vi "Send_Datagram.vi"() -> ()   [LabVIEW 2018]
uses:
  Type_Def/Type_Def ControlState.ctl
panel:
  in  "Port Number":u16
  in  "IP Address target":string
  in  "Team ID":u8
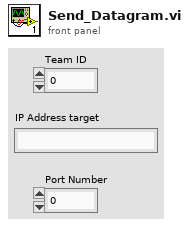
[diagram p1: front panel]
types:
  T1 = typedef "Type_Def ControlState.ctl" = enum16{"Blank", "Systems Check", "Idle", "Ready", "Pushing", "CrawlingPrecharge", "Braking", "Fault", "Boot Up", "Unpowered", "Crawling", "Shutdown", "Service Push", "Service Wait", "Vent", "Precharge"}
  T2 = cluster{"Forward":bool, "Low Side":bool, "Precharge":bool, "High Side":bool, "Digital Out 5":bool, "Digital Out 6":bool, "Digital Out 7 ":bool, "24 Power":bool, "Tank Valve ":bool, "Brake Valve":bool, "Pump":bool, "Digital Out 1 ":bool, "Digital Out 2":bool, "Digital Out 3":bool, "Digital Out 4 ":bool, "Reverse":bool}
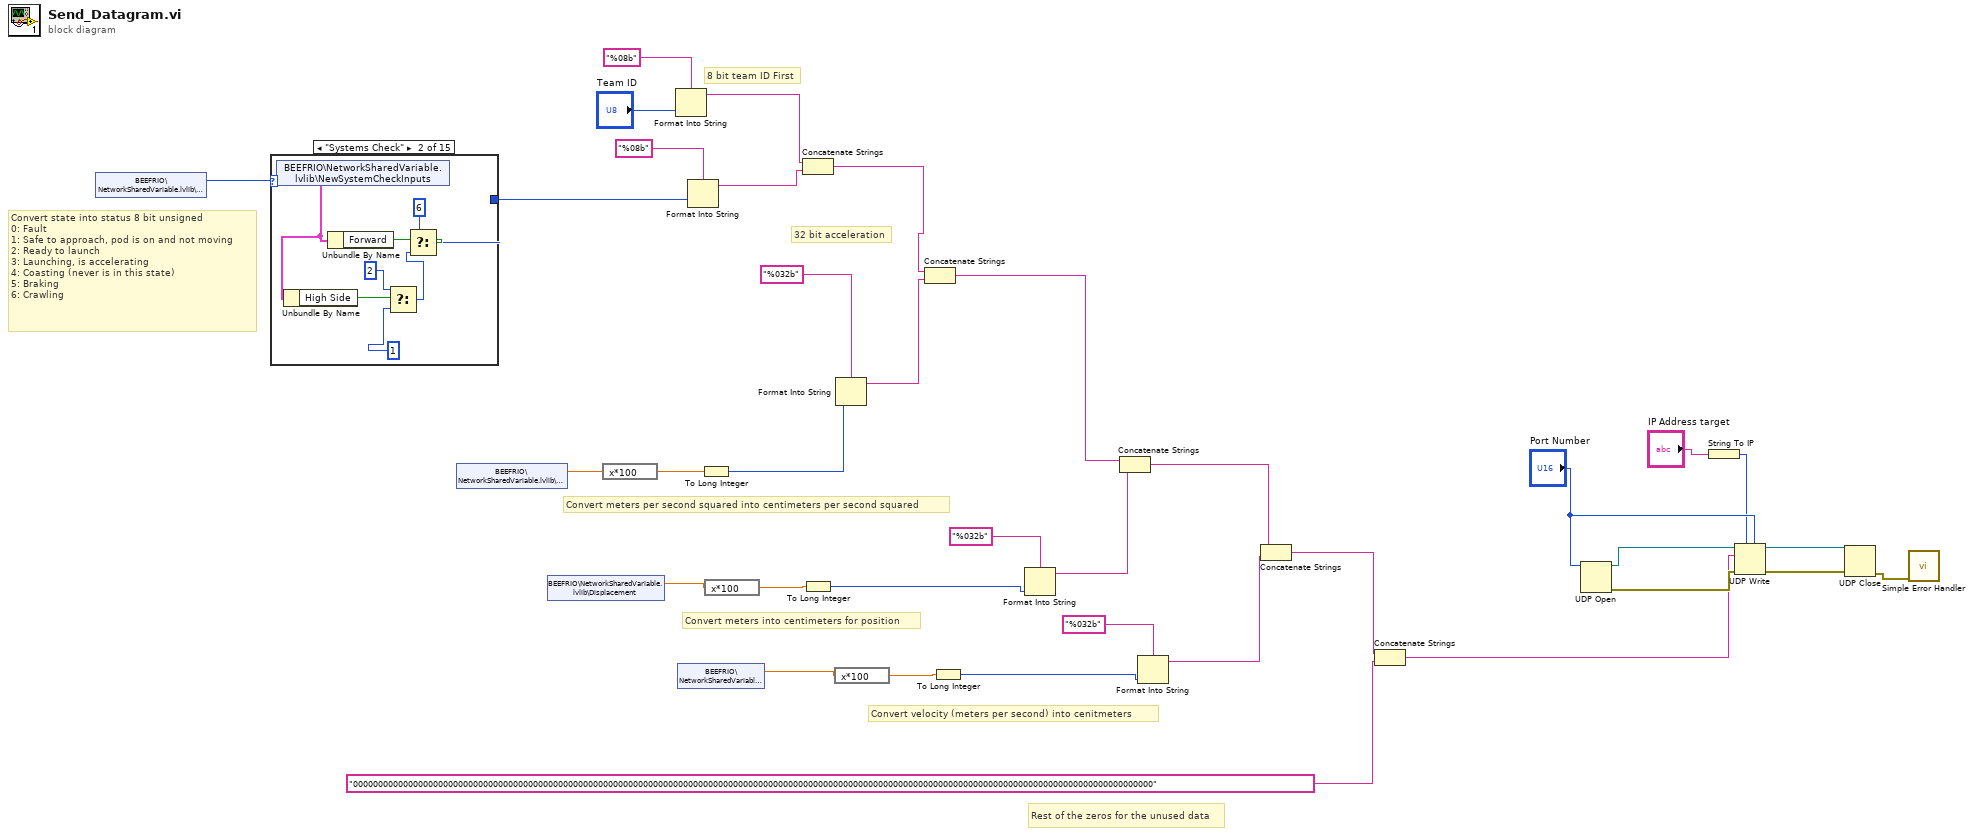
[diagram p0: block diagram]
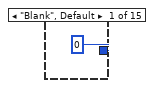
[diagram p2: hidden frame]
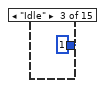
[diagram p3: hidden frame]
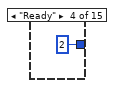
[diagram p4: hidden frame]
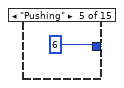
[diagram p5: hidden frame]
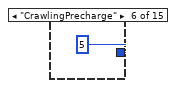
[diagram p6: hidden frame]
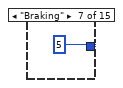
[diagram p7: hidden frame]
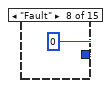
[diagram p8: hidden frame]
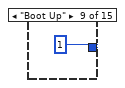
[diagram p9: hidden frame]
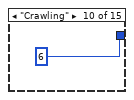
[diagram p10: hidden frame]
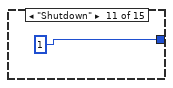
[diagram p11: hidden frame]
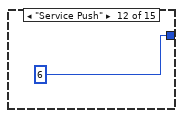
[diagram p12: hidden frame]
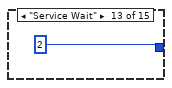
[diagram p13: hidden frame]
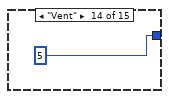
[diagram p14: hidden frame]
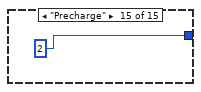
[diagram p15: hidden frame]
diagram:
  # "Rest of the zeros for the unused data"
  # "Convert velocity (meters per second) into cenitmeters"
  # "Convert meters into centimeters for position"
  # "32 bit acceleration"
  # "Convert meters per second squared into centimeters per second squared"
  # "8 bit team ID First"
  # "Convert state into status 8 bit unsigned\n0: Fault\n1: Safe to approach, pod is on and not moving\n2: Ready to launch\n3: Launching, is accelerating\n4: Coasting (never is in this state)\n5: Braking\n6: Crawling"
  n1 = shared-variable "BEEFRIO\\NetworkSharedVariable.lvlib\\CurrentState"() -> (w2:T1)  [unwired: 1 in, 1 out]
  n2 = case shown="\"Systems Check\"" w2 {
    tunnel: [u8 0 w38 u8 1 u8 2 u8 6 u8 5 u8 5 u8 0 u8 1 u8 6 u8 1 u8 6 u8 2 u8 5 u8 2] -> w1
    frame "Blank", Default {
    }
    frame "Systems Check" {
      n3 = shared-variable "BEEFRIO\\NetworkSharedVariable.lvlib\\NewSystemCheckInputs"() -> (w43:T2)  [unwired: 1 in, 1 out]
      n4 = Unbundle By Name(w43) -> ("High Side"=w42:bool)
      n5 = Unbundle By Name(w43) -> ("Forward"=w45:bool)
      n6 = Select(t=u8 2, s=w42, f=u8 1) -> (s? t:f=w39:u8)
      n7 = Select(t=u8 6, s=w45, f=w39) -> (s? t:f=w38:u8)
    }
    frame "Idle" {
    }
    frame "Ready" {
    }
    frame "Pushing" {
    }
    frame "CrawlingPrecharge" {
    }
    frame "Braking" {
    }
    frame "Fault" {
    }
    frame "Boot Up" {
    }
    frame "Crawling" {
    }
    frame "Shutdown" {
    }
    frame "Service Push" {
    }
    frame "Service Wait" {
    }
    frame "Vent" {
    }
    frame "Precharge" {
    }
  }
  n8 = shared-variable "BEEFRIO\\NetworkSharedVariable.lvlib\\Acceleration"() -> (w8:dbl)  [unwired: 1 in, 1 out]
  n9 = shared-variable "BEEFRIO\\NetworkSharedVariable.lvlib\\Displacement"() -> (w11:dbl)  [unwired: 1 in, 1 out]
  n10 = expression code="x*100"(w8) -> (w7:dbl)
  n11 = Format Into String(format string="%08b", "Team ID") -> (resulting string=w33:string)  [unwired: 2 in, 1 out]
  n12 = shared-variable "BEEFRIO\\NetworkSharedVariable.lvlib\\Velocity"() -> (w5:dbl)  [unwired: 1 in, 1 out]
  n13 = Format Into String(format string="%08b", w1) -> (resulting string=w35:string)  [unwired: 2 in, 1 out]
  n14 = To Long Integer(number=w7) -> (32bit integer=w6:i32)
  n15 = expression code="x*100"(w11) -> (w10:dbl)
  n16 = Concatenate Strings(w33, w35) -> (w30:string)
  n17 = To Long Integer(number=w10) -> (32bit integer=w9:i32)
  n18 = expression code="x*100"(w5) -> (w4:dbl)
  n19 = Format Into String(format string="%032b", w6) -> (resulting string=w29:string)  [unwired: 2 in, 1 out]
  n20 = Concatenate Strings(w30, w29) -> (w26:string)
  n21 = To Long Integer(number=w4) -> (32bit integer=w3:i32)
  n22 = Format Into String(format string="%032b", w9) -> (resulting string=w27:string)  [unwired: 2 in, 1 out]
  n23 = Concatenate Strings(w26, w27) -> (w23:string)
  n24 = Format Into String(format string="%032b", w3) -> (resulting string=w24:string)  [unwired: 2 in, 1 out]
  n25 = Concatenate Strings(w23, w24) -> (w21:string)
  n26 = Concatenate Strings(w21, "0000000000000000000000000000000000000000000000000000000000000000000000000000000000000000000000000000000000000000000000000000000000000000000000000000000000000000") -> (w13:string)
  n27 = UDP Open(11:"Port Number") -> (port=w19:refnum<k16>, 0:w17:errorcluster)  [unwired: 4 in, 1 out]
  n28 = String To IP(1:"IP Address target") -> (0:w12:u32)
  n29 = UDP Write(address=w12, port or service name="Port Number", connection ID=w19, data in=w13, 8:w17) -> (error out=w16:errorcluster, 3:w18:refnum<k16>)  [unwired: 1 in]
  n30 = UDP Close(connection ID=w18, 8:w16) -> (error out=w15:errorcluster)  [unwired: 1 out]
  n31 = call <vilib>:"Simple Error Handler.vi"("error in (no error)"=w15) -> ()  [unwired: 4 in, 5 out]
